vi "Get Sheet Names.vi"(8 "error IO":errorcluster, 11 "ooCalc in":refnum<class "ooCalc.lvclass">) -> (0 "error out":errorcluster, 2 "Sheets":string[](array[string]), 3 "ooCalc out":refnum<class "ooCalc.lvclass">)   [LabVIEW 2009, in "ooCalc.lvclass"]
uses:
  ooCalc.lvclass
  C:/Projets/LAVAG/OpenOfficeRGT/AODL/DLLs/AODL.dll
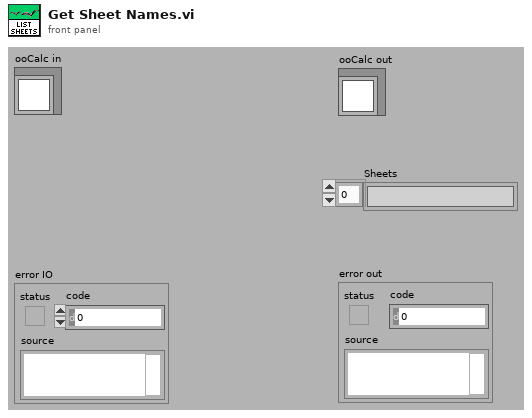
[diagram p1: front panel]
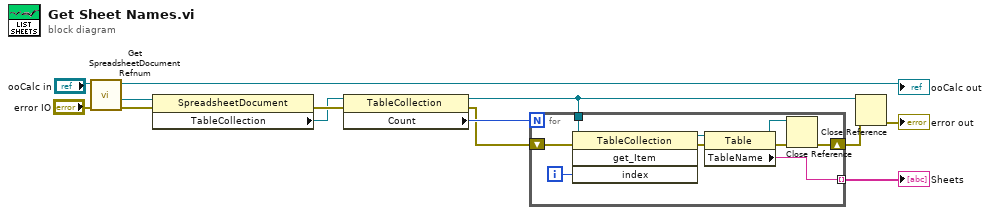
[diagram p0: block diagram]
diagram:
  n1 = call-dynamic "Get SpreadsheetDocument Refnum.vi"("error in (no error)"="error IO", "ooCalc in"="ooCalc in") -> ("error out"=w2:errorcluster, "SpreadsheetDocument"=w1:refnum<k24>, "ooCalc out"=→"ooCalc out":refnum<class "ooCalc.lvclass">)  [unwired: 7 in]
  n2 = property class="SpreadsheetDocument"(reference=w1, error in=w2) -> (error out=w12:errorcluster, "TableCollection"=w10:refnum<k24>)  [unwired: 1 out]
  n3 = property class="TableCollection"(reference=w10, error in=w12) -> (reference out=w8:refnum<k24>, error out=w7:errorcluster, "Count"=w9:i32)
  n4 = for {
    N: w9 -> [_]
    tunnel: [w19] -> w11 mode=indexing
    tunnel: w8 -> [w17]
    shift-right: [w15] -> w6
    shift-left: w7 -> [w16]
    i -> [w22]
    n5 = invoke class="TableCollection" method="get_Item"(reference=w17, error in=w16, "index"=w22) -> (error out=w21:errorcluster, "get_Item"=w20:refnum<k24>)  [unwired: 1 in, 2 out]
    n6 = property class="Table"(reference=w20, error in=w21) -> (reference out=w18:refnum<k24>, error out=w14:errorcluster, "TableName"=w19:string)
    n7 = Close Reference(reference=w18, error in (no error)=w14) -> (error out=w15:errorcluster)
  }
  "Sheets" <- w11
  n8 = Close Reference(reference=w8, error in (no error)=w6) -> (error out=→"error out":errorcluster)
